vi "CPP-PowerLawFit.vi"() -> (0 "New Values In":string[][](array[string])=[["Test data5"]], 1 "New Chs In":string[](array[string])=["30-10-03:New:Channel new5"])   [LabVIEW 2013]
uses:
  Results_plotter_Global.vi
panel:
  in  "Zref":dbl
  in  "Fit Zmax":dbl
  in  "Fit Zmin":dbl
  # "This VI receives \"classic\" transposed plots of U/Uref vs Z, and fits a power law to them over the range specified on this front panel, for the stated Zref- which will be normalised to internally here.\nBest to do some trial runs to establish a sensible fit range, and then batch process profiles which share common fit ranges."
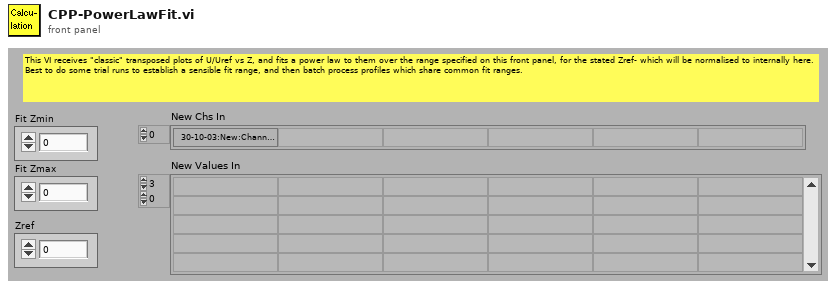
[diagram p1: front panel]
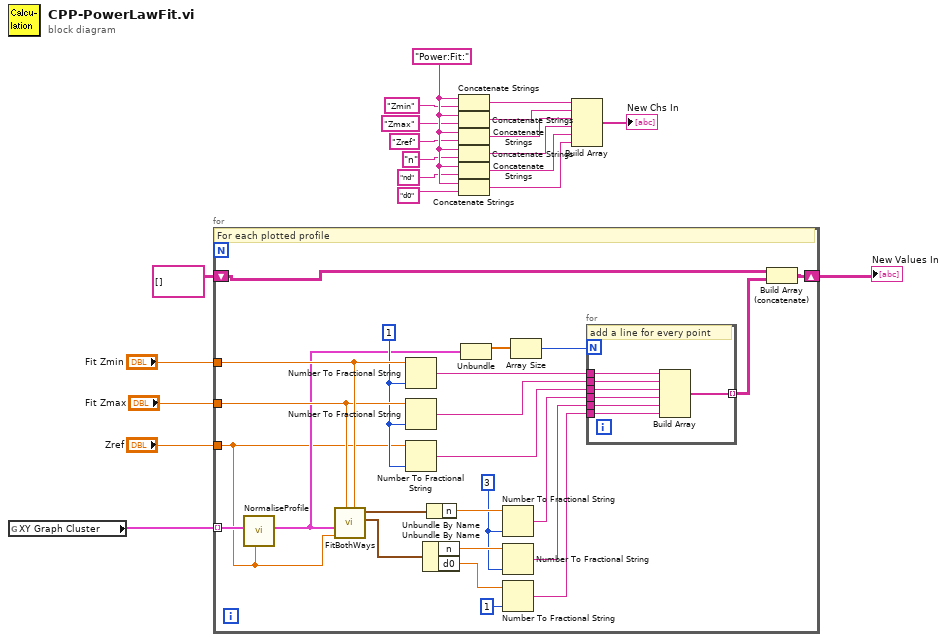
[diagram p0: block diagram]
diagram:
  w13 = "Power:Fit:"
  n1 = global read "Results_plotter_Global.vi" "XY Graph Cluster"() -> (w3:cluster{dbl[], dbl[]}[])
  n2 = for {
    tunnel: "Fit Zmin" -> [w42]
    tunnel: "Fit Zmax" -> [w41]
    tunnel: "Zref" -> [w21]
    tunnel: w3 -> [w23] mode=indexing
    shift-right: [w28] -> w1
    shift-left: string[][] [] -> [w27]
    w36 = i16 3 ("precision (6)")
    w40 = i16 1 ("precision (6)")
    # "For each plotted profile"
    n3 = call "NormaliseProfile.vi"("Zref"=w21, "zUCluster"=w23) -> ("zUCluster 2"=w22:cluster{dbl[], dbl[]})  [unwired: 9 in]
    n4 = call "FitBothWays.vi"("Fit Zmin"=w42, "Fit Zmax"=w41, "Zref"=w21, "zUCluster in"=w22) -> ("PowerLawWithDisplacement"=w43:cluster{"n":dbl, "d0":dbl}, "PowerLawNoDisplacement"=w44:cluster{"n":dbl, "d0":dbl})  [unwired: 6 in]
    n5 = Number To Fractional String(number=w42, precision (6)=w40) -> (F-format string=w34:string)  [unwired: 2 in]
    n6 = Number To Fractional String(number=w41, precision (6)=w40) -> (F-format string=w33:string)  [unwired: 2 in]
    n7 = Number To Fractional String(number=w21, precision (6)=w40) -> (F-format string=w32:string)  [unwired: 2 in]
    n8 = Unbundle By Name(w43) -> ("n"=w38:dbl, "d0"=w37:dbl)
    n9 = Unbundle By Name(w44) -> ("n"=w39:dbl)
    n10 = Unbundle(w22) -> (w25:dbl[])  [unwired: 1 out]
    n11 = Number To Fractional String(number=w39, precision (6)=w36) -> (F-format string=w31:string)  [unwired: 2 in]
    n12 = Number To Fractional String(number=w38, precision (6)=w36) -> (F-format string=w30:string)  [unwired: 2 in]
    n13 = Number To Fractional String(number=w37, precision (6)=i16 1) -> (F-format string=w29:string)  [unwired: 2 in]
    n14 = Array Size(array=w25) -> (size(s)=w26:i32)
    n15 = for {
      N: w26 -> [_]
      tunnel: w34 -> [w51]
      tunnel: w33 -> [w50]
      tunnel: w32 -> [w49]
      tunnel: w31 -> [w48]
      tunnel: w30 -> [w47]
      tunnel: w29 -> [w46]
      tunnel: [w45] -> w24 mode=indexing
      # "add a line for every point"
      n16 = Build Array(w51, w50, w49, w48, w47, w46) -> (w45:string[])
    }
    n17 = Build Array (concatenate)(w27, w24) -> (w28:string[][])
  }
  "New Values In" <- w1
  n18 = Concatenate Strings(w13, "Zmin" ("string")) -> (w19:string)
  n19 = Concatenate Strings(w13, "Zmax" ("string")) -> (w18:string)
  n20 = Concatenate Strings(w13, "Zref" ("string")) -> (w17:string)
  n21 = Concatenate Strings(w13, "n" ("string")) -> (w16:string)
  n22 = Concatenate Strings(w13, "nd" ("string")) -> (w15:string)
  n23 = Concatenate Strings(w13, "d0" ("string")) -> (w14:string)
  n24 = Build Array(w19, w18, w17, w16, w15, w14) -> (→"New Chs In":string[])
